vi "Build Time to Next Message.vi"(7 "Virtual Memory Unit in":refnum<class "Virtual Memory Unit.lvclass">, 8 "error in (no error)":errorcluster, 10 "Starting Address":u16 format="%04x", 11 "Message in":refnum<class "Message.lvclass">) -> (0 "error out":errorcluster, 2 "Next Available Address":u16 format="%04x", 3 "Message out":refnum<class "Message.lvclass">, 5 "Virtual Memory Unit out":refnum<class "Virtual Memory Unit.lvclass">)   [LabVIEW 2020, in "BCI-1553 API.lvlib" / "Message.lvclass"]
doc: "Writes the Time to Next Message value into memory. This value determines the amount of time the execution will halt before sending out the the next message."
uses:
  Message.lvclass
  Dependencies/Virtual Memory Unit/Virtual Memory Unit.lvclass
  Message.lvclass/Message.ctl
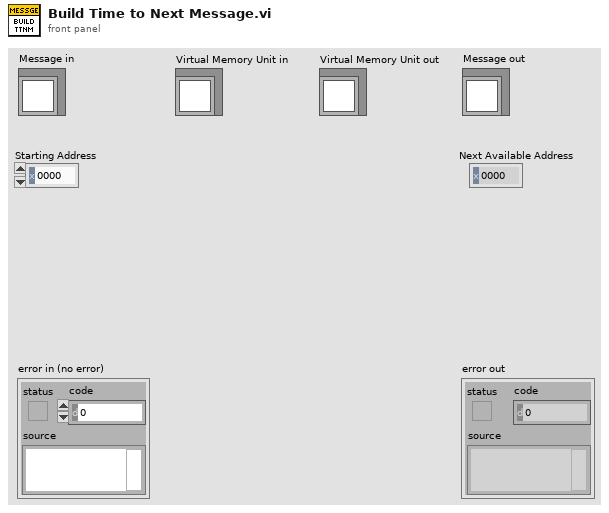
[diagram p1: front panel]
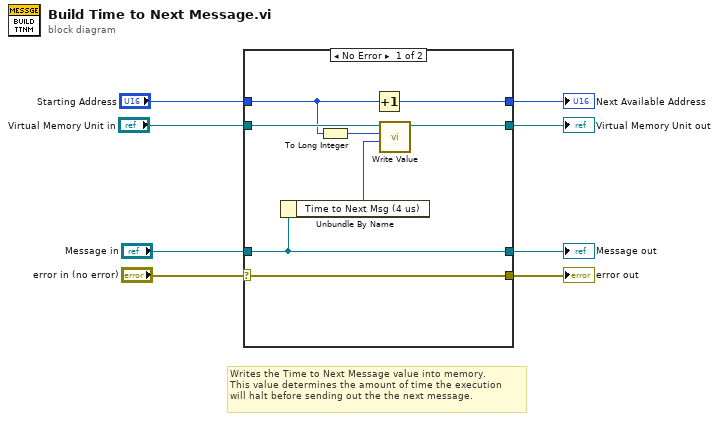
[diagram p0: block diagram]
diagram:
  # "Writes the Time to Next Message value into memory.\nThis value determines the amount of time the execution\nwill halt before sending out the the next message."
  n1 = case shown="No Error" "error in (no error)" {
    selector: "error in (no error)" -> [w16 w20]
    tunnel: [w16 w20] -> w7
    tunnel: [w15 w19] -> w5
    tunnel: "Message in" -> [w15 w19]
    tunnel: "Virtual Memory Unit in" -> [w13 w18]
    tunnel: [w12 w18] -> w3
    tunnel: [w14 w17] -> w2
    tunnel: "Starting Address" -> [w10 w17]
    frame No Error {
      n2 = Unbundle By Name(w15) -> ("Time to Next Msg (4 us)"=w9:u16)
      n3 = To Long Integer(number=w10) -> (32bit integer=w11:i32)
      n4 = Increment(x=w10) -> (x+1=w14:u16)
      n5 = call "Write Value.vi"("Value"=w9, "Index"=w11, "Virtual Memory Unit in"=w13) -> ("Virtual Memory Unit out"=w12:refnum<class "Virtual Memory Unit.lvclass">)  [unwired: 7 in, 1 out]
    }
    frame Error {
    }
  }
  "error out" <- w7
  "Message out" <- w5
  "Virtual Memory Unit out" <- w3
  "Next Available Address" <- w2
